vi "Fetch (Limit).vi"(8 "error in (no error)":errorcluster, 11 "VISA resource name":refnum<visa-resource-name>) -> (0 "error out":errorcluster, 1 "Upper Limit Failure Count":dbl, 2 "Lower Limit Failure Count":dbl, 3 "VISA resource name out":refnum<visa-resource-name>, 4 "Total  Failure Count":dbl, 5 "Limit Status":bool, 6 "Total  Pass Count":dbl)   [LabVIEW 2020, in "Counter.lvlib" / "PICOTEST U62XXA series.lvlib"]
doc: "Queries and returns the results of the Limit test.\n\n<B>Note:</B>\n\nIf no valid result exists, 0 is returned."
uses:
  PICOTEST U62XXA series.lvlib
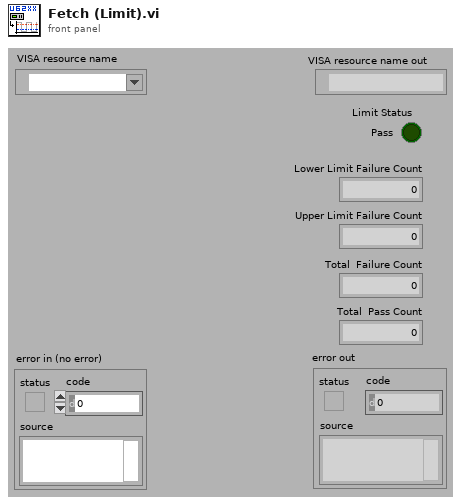
[diagram p1: front panel]
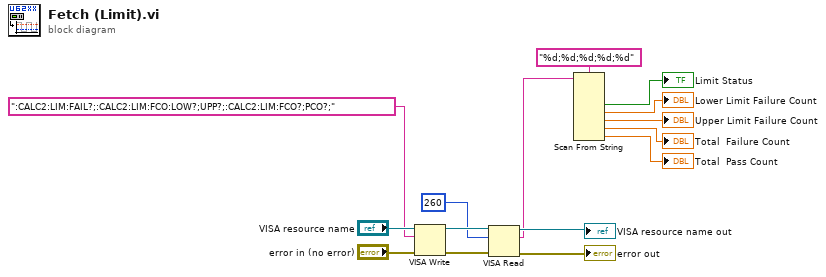
[diagram p0: block diagram]
diagram:
  n1 = VISA Write(VISA resource name="VISA resource name", write buffer=":CALC2:LIM:FAIL?;:CALC2:LIM:FCO:LOW?;UPP?;:CALC2:LIM:FCO?;PCO?;" ("format string"), error in (no error)="error in (no error)") -> (VISA resource name out=w13:refnum<visa-resource-name>, error out=w12:errorcluster)  [unwired: 1 out]
  n2 = VISA Read(VISA resource name=w13, byte count=u32 260, error in (no error)=w12) -> (VISA resource name out=→"VISA resource name out":refnum<visa-resource-name>, read buffer=w8:string, error out=→"error out":errorcluster)  [unwired: 1 out]
  n3 = Scan From String(format string="%d;%d;%d;%d;%d", input string=w8) -> (output 1=→"Limit Status":bool, output 2=→"Lower Limit Failure Count":dbl, output 3=→"Upper Limit Failure Count":dbl, output 4=→"Total  Failure Count":dbl, output 5=→"Total  Pass Count":dbl)  [unwired: 7 in, 3 out]
